vi "ProcessName.vi"() -> (1 "process name":string="DataEventCreator")   [LabVIEW 2017, in "DataEventCreator.lvlib"]
uses:
  <vilib>/addons/InsightCM/Devices/Shared/Common/DataEventCreator/DataEventCreator.lvlib
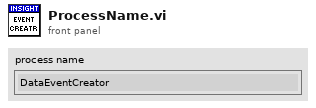
[diagram p1: front panel]
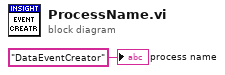
[diagram p0: block diagram]
diagram:
  "process name" <- "DataEventCreator" ("ProcessName")
